vi "DAQmx_SyncAll.vi"(8 "error in (no error)":errorcluster, 11 "Array in":refnum<class "DAQmx.lvclass">[](array[class])) -> (0 "error out":errorcluster, 3 "Array out":refnum<class "DAQmx.lvclass">[](array[class]))   [LabVIEW 2016, in "DAQmx.lvclass"]
uses:
  DAQmx.lvclass
  DAQmx.lvclass/DAQmx.ctl
  <vilib>/DAQmx/configure/trigger.llb/DAQmx Start Trigger (Digital Edge).vi
  <resource>/objmgr/daqmx.rc
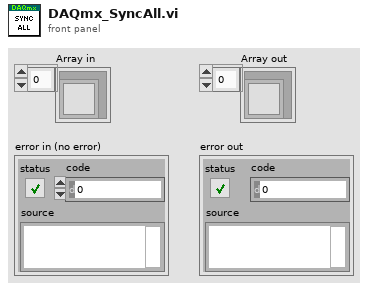
[diagram p1: front panel]
types:
  T1 = typedef "DAQmx.lvclass/DAQmx.Config.ctl" = cluster{"Buffer Size (S)":i32, "Master Slave":enum16{"MASTER", "SLAVE"}}
  T2 = cluster{"RefClk.Src":tag, "SyncPulse.src":tag, "StartTrigger.src":tag, "SyncPulse.SyncTime":dbl}
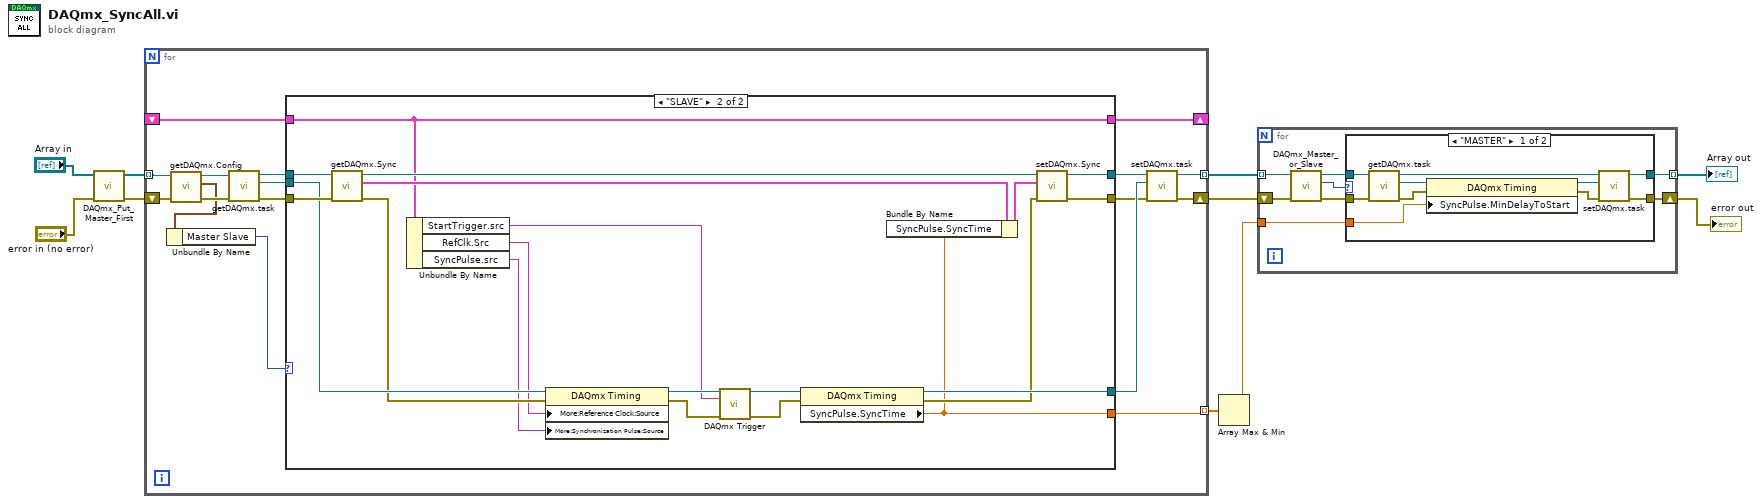
[diagram p0: block diagram]
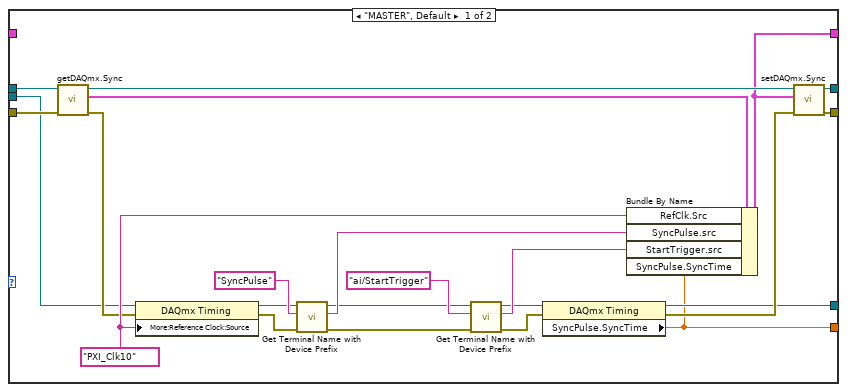
[diagram p2: hidden frame]
diagram:
  n1 = call "DAQmx_Put_Master_First.vi"("error in (no error)"="error in (no error)", "DAQmx in"="Array in") -> ("error out"=w1:errorcluster, "DAQmx out"=w2:refnum<class "DAQmx.lvclass">[])  [unwired: 8 in]
  n2 = for {
    tunnel: w2 -> [w16] mode=indexing
    shift-right: [w21] -> w7
    shift-left: w1 -> [w13]
    tunnel: [w20] -> w8 mode=indexing
    tunnel: [w19] -> w6 mode=indexing
    shift-right: [w18] -> _
    shift-left: _ -> [w17]
    n3 = call "getDAQmx.Config.vi"("error in (no error)"=w13, "DAQmx in"=w16) -> ("error out"=w14:errorcluster, "DAQmx.Config"=w12:T1, "DAQmx out"=w15:refnum<class "DAQmx.lvclass">)  [unwired: 7 in]
    n4 = Unbundle By Name(w12) -> ("Master Slave"=w11:enum16{"MASTER", "SLAVE"})
    n5 = call "getDAQmx.task.vi"("error in (no error)"=w14, "DAQmx in"=w15) -> ("error out"=w23:errorcluster, "task"=w27:refnum<k21>, "DAQmx out"=w25:refnum<class "DAQmx.lvclass">)  [unwired: 7 in]
    n6 = case shown="\"SLAVE\"" w11 {
      tunnel: w27 -> [w32 w66]
      tunnel: [w30 w54] -> w26
      tunnel: w23 -> [w36 w67]
      tunnel: w25 -> [w39 w70]
      tunnel: [w37 w69] -> w24
      tunnel: [w33 w56] -> w22
      tunnel: [w28 w51] -> w20
      tunnel: [w29 w52] -> w18
      tunnel: w17 -> [_ w52]
      frame "MASTER", Default {
        w41 = tag "PXI_Clk10" ("RefClk.Src")
        n7 = call "getDAQmx.Sync.vi"("error in (no error)"=w36, "DAQmx in"=w39) -> ("error out"=w35:errorcluster, "Sync"=w34:T2, "DAQmx out"=w38:refnum<class "DAQmx.lvclass">)  [unwired: 7 in]
        n8 = property class="DAQmx Timing"(reference=w32, error in=w35, "More:Reference Clock:Source"=w41) -> (reference out=w48:refnum<k21>, error out=w47:errorcluster)
        n9 = call "Get Terminal Name with Device Prefix.vi"("error in (no error)"=w47, "Local Terminal Name"="SyncPulse", "task/channels in"=w48) -> ("error out"=w44:errorcluster, "Terminal Name with Device Prefix"=w46:tag, "task out"=w45:refnum<k21>)  [unwired: 6 in]
        n10 = call "Get Terminal Name with Device Prefix.vi"("error in (no error)"=w44, "Local Terminal Name"="ai/StartTrigger", "task/channels in"=w45) -> ("error out"=w40:errorcluster, "Terminal Name with Device Prefix"=w43:tag, "task out"=w42:refnum<k21>)  [unwired: 6 in]
        n11 = property class="DAQmx Timing"(reference=w42, error in=w40) -> (reference out=w30:refnum<k21>, error out=w31:errorcluster, "SyncPulse.SyncTime"=w28:dbl)
        n12 = Bundle By Name(cluster=w34, "RefClk.Src"=w41, "SyncPulse.src"=w46, "StartTrigger.src"=w43, "SyncPulse.SyncTime"=w28) -> (w29:T2)
        n13 = call "setDAQmx.Sync.vi"("error in (no error)"=w31, "Sync"=w29, "DAQmx in"=w38) -> ("error out"=w33:errorcluster, "DAQmx out"=w37:refnum<class "DAQmx.lvclass">)  [unwired: 7 in]
      }
      frame "SLAVE" {
        n14 = call "getDAQmx.Sync.vi"("error in (no error)"=w67, "DAQmx in"=w70) -> ("error out"=w65:errorcluster, "Sync"=w57:T2, "DAQmx out"=w68:refnum<class "DAQmx.lvclass">)  [unwired: 7 in]
        n15 = Unbundle By Name(w52) -> ("StartTrigger.src"=w55:tag, "RefClk.Src"=w60:tag, "SyncPulse.src"=w59:tag)
        n16 = property class="DAQmx Timing"(reference=w66, error in=w65, "More:Reference Clock:Source"=w60, "More:Synchronization Pulse:Source"=w59) -> (reference out=w63:refnum<k21>, error out=w64:errorcluster)
        n17 = call-poly <vilib>:"DAQmx Trigger.vi"("task/channels in"=w63, "source"=w55, "error in"=w64) -> ("task out"=w62:refnum<k21>, "error out"=w61:errorcluster)  [unwired: 11 in]
        n18 = property class="DAQmx Timing"(reference=w62, error in=w61) -> (reference out=w54:refnum<k21>, error out=w53:errorcluster, "SyncPulse.SyncTime"=w51:dbl)
        n19 = Bundle By Name(cluster=w57, "SyncPulse.SyncTime"=w51) -> (w58:T2)
        n20 = call "setDAQmx.Sync.vi"("error in (no error)"=w53, "Sync"=w58, "DAQmx in"=w68) -> ("error out"=w56:errorcluster, "DAQmx out"=w69:refnum<class "DAQmx.lvclass">)  [unwired: 7 in]
      }
    }
    n21 = call "setDAQmx.task.vi"("error in (no error)"=w22, "task"=w26, "DAQmx in"=w24) -> ("error out"=w21:errorcluster, "DAQmx out"=w19:refnum<class "DAQmx.lvclass">)  [unwired: 7 in]
  }
  n22 = Array Max & Min(array=w8) -> (max value=w5:dbl)  [unwired: 3 out]
  n23 = for {
    tunnel: w5 -> [w73]
    tunnel: w6 -> [w78] mode=indexing
    tunnel: [w72] -> w10 mode=indexing
    shift-right: [w71] -> w9
    shift-left: w7 -> [w77]
    n24 = call "DAQmx_Master_or_Slave.vi"("error in (no error)"=w77, "DAQmx in"=w78) -> ("error out"=w74:errorcluster, "Enum"=w76:enum16{"MASTER", "SLAVE"}, "DAQmx out"=w75:refnum<class "DAQmx.lvclass">)  [unwired: 7 in]
    n25 = case shown="\"MASTER\"" w76 {
      tunnel: w75 -> [w88 w90]
      tunnel: w74 -> [w87 w89]
      tunnel: w73 -> [w83 _]
      tunnel: [w81 w90] -> w72
      tunnel: [w80 w89] -> w71
      frame "MASTER" {
        n26 = call "getDAQmx.task.vi"("error in (no error)"=w87, "DAQmx in"=w88) -> ("error out"=w79:errorcluster, "task"=w86:refnum<k21>, "DAQmx out"=w84:refnum<class "DAQmx.lvclass">)  [unwired: 7 in]
        n27 = property class="DAQmx Timing"(reference=w86, error in=w79, "SyncPulse.MinDelayToStart"=w83) -> (reference out=w85:refnum<k21>, error out=w82:errorcluster)
        n28 = call "setDAQmx.task.vi"("error in (no error)"=w82, "task"=w85, "DAQmx in"=w84) -> ("error out"=w80:errorcluster, "DAQmx out"=w81:refnum<class "DAQmx.lvclass">)  [unwired: 7 in]
      }
      frame "SLAVE", Default {
      }
    }
  }
  "error out" <- w9
  "Array out" <- w10
